vi "Start.vi"(0 "On/Off":bool, 1 "Control in":T1={"queue"=refnum, "error"={"status"=FALSE, "code"=0, "source"=""}, "Step"={"Name"="", "Timeout"=0.0}, "Algorythm"=[{"Name"="Init", "Timeout"=0.0}]}) -> (15 "Control out":T1={"queue"=refnum, "error"={"status"=FALSE, "code"=0, "source"=""}, "Step"={"Name"="", "Timeout"=0.0}, "Algorythm"=[{"Name"="Init", "Timeout"=0.0}]})   [LabVIEW 2018, in "SFC.lvlib"]
uses:
  SFC.lvlib
  TypeDef/Control TypeDef.ctl
  TypeDef/Step TypeDef.ctl
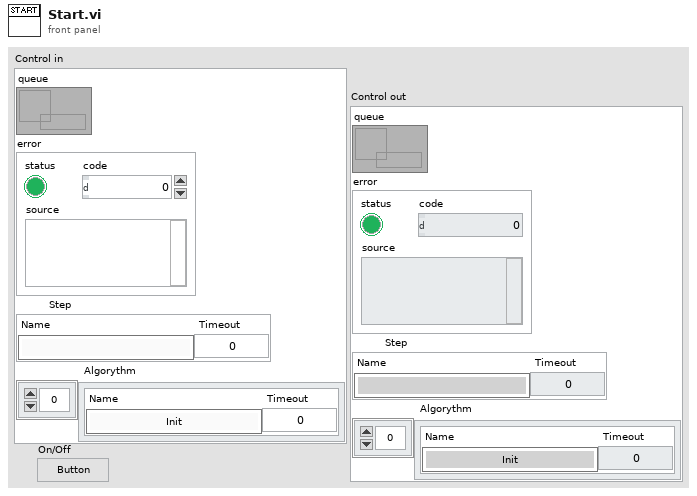
[diagram p1: front panel]
types:
  T1 = typedef "SFC.lvlib/Control TypeDef.ctl" = cluster{"queue":refnum<queue>, "error":errorcluster, "Step":T2, "Algorythm":T2[]}
  T2 = typedef "SFC.lvlib/Step TypeDef.ctl" = cluster{"Name":string, "Timeout":dbl}
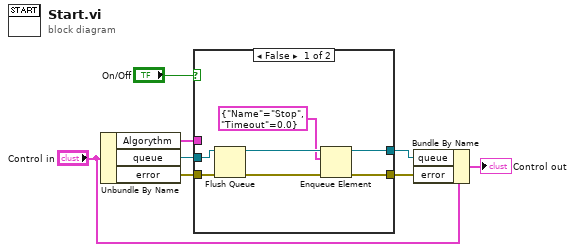
[diagram p0: block diagram]
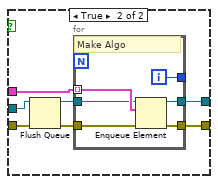
[diagram p2: hidden frame]
diagram:
  n1 = Unbundle By Name("Control in") -> ("Algorythm"=w1:T2[], "queue"=w7:refnum<queue>, "error"=w6:errorcluster)
  n2 = case shown="False" "On/Off" {
    tunnel: w7 -> [w15 w22]
    tunnel: w6 -> [w14 w21]
    tunnel: [w10 w18] -> w3
    tunnel: [w9 w17] -> w2
    tunnel: w1 -> [_ w16]
    frame False {
      n3 = Flush Queue(queue=w15, error in (no error)=w14) -> (queue out=w13:refnum<queue>, error out=w12:errorcluster)  [unwired: 1 out]
      n4 = Enqueue Element(queue=w13, element=T2 {"Name"="Stop", "Timeout"=0.0}, error in (no error)=w12) -> (queue out=w10:refnum<queue>, error out=w9:errorcluster)  [unwired: 1 in, 1 out]
    }
    frame True {
      n5 = Flush Queue(queue=w22, error in (no error)=w21) -> (queue out=w20:refnum<queue>, error out=w19:errorcluster)  [unwired: 1 out]
      n6 = for {
        tunnel: w16 -> [w28] mode=indexing
        tunnel: w20 -> [w27]
        tunnel: w19 -> [w26]
        tunnel: [w25] -> _
        tunnel: [w24] -> w18
        tunnel: [w23] -> w17
        i -> [w25]
        # "Make Algo"
        n7 = Enqueue Element(queue=w27, element=w28, error in (no error)=w26) -> (queue out=w24:refnum<queue>, error out=w23:errorcluster)  [unwired: 1 in, 1 out]
      }
    }
  }
  n8 = Bundle By Name(cluster="Control in", "queue"=w3, "error"=w2) -> (→"Control out":T1)
